vi "ConfigInstr.vi"(6 "InstrumentName":string, 7 "VisaRessIn":refnum<visa-resource-name>, 8 "error in (no error)":errorcluster caption="entrée d'erreur (pas d'erreur)", 9 "FirstClassInst":bool, 10 "Function":string, 11 "GenData In":refnum<class "Calculations.lvclass"> caption="DNL_LabVIEW Object in") -> (0 "error out":errorcluster caption="sortie d'erreur", 3 "GenData Out":refnum<class "Calculations.lvclass"> caption="DNL_LabVIEW Object out")   [LabVIEW 2019, in "Calculations.lvclass"]
uses:
  Calculations.lvclass
  C:/Programmes Labview/LabScanV1A/DevicesClass/BaseDevice/BaseDevice.lvclass
  DefaultDev_Func.ctl
  Calculations.lvclass/Calculations.ctl
  DevicesClass/BaseDevice/BaseDevice.lvclass/BaseDevice.ctl
  DevicesClass/BaseDevice/Accessor/SetShowInstrNm.vi
panel:
  in  "Class_Func":T1
  out "VisaRessOut":refnum<visa-resource-name>
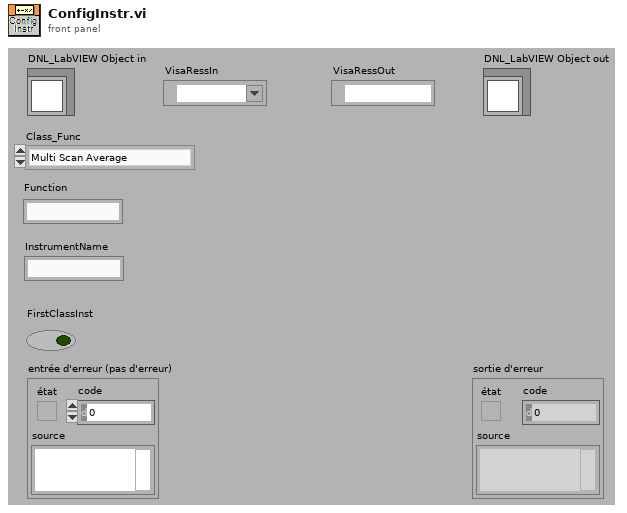
[diagram p1: front panel]
types:
  T1 = typedef "Calculations.lvclass/DefaultDev_Func.ctl" = enum16{"Multi Scan Average", "Running Average", "Summ"}
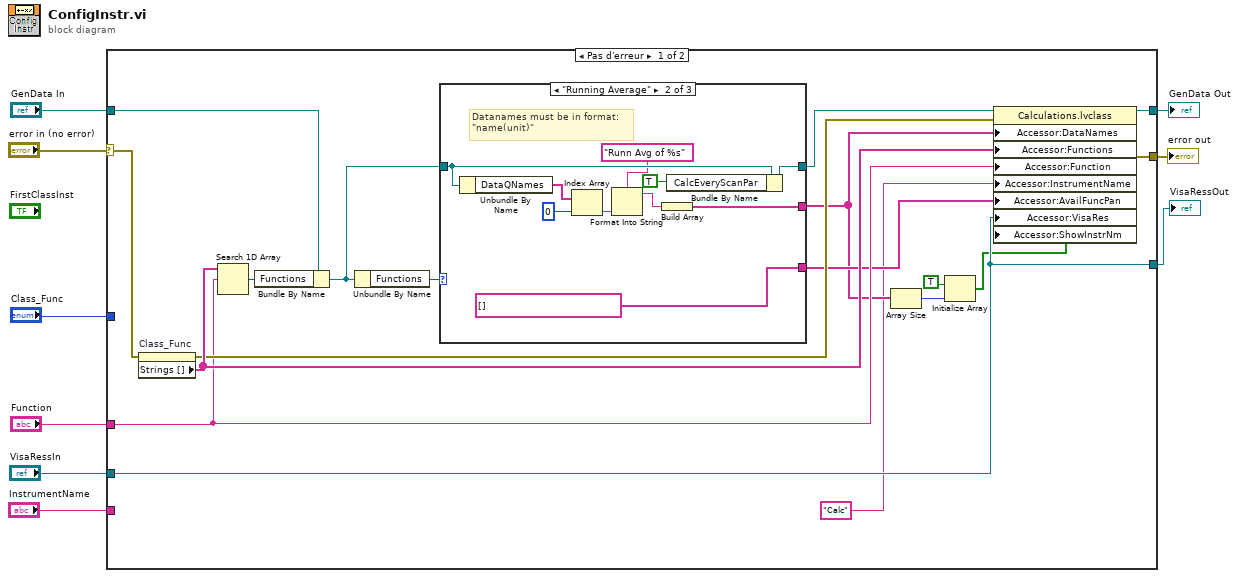
[diagram p0: block diagram]
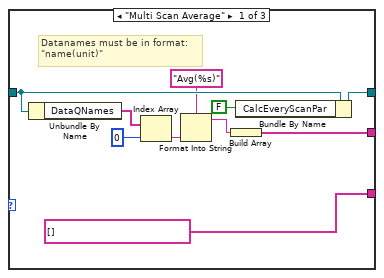
[diagram p2: hidden frame]
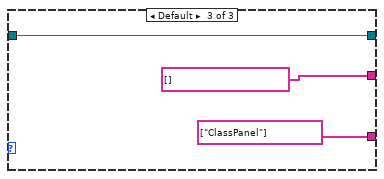
[diagram p3: hidden frame]
diagram:
  n1 = case shown="Pas d'erreur" "error in (no error)" {
    selector: "error in (no error)" -> [w21 w52]
    tunnel: [w27 w52] -> w8
    tunnel: "GenData In" -> [w22 w51]
    tunnel: [w26 w51] -> w6
    tunnel: "Class_Func" -> [_ _]
    tunnel: "Function" -> [w17 _]
    tunnel: "InstrumentName" -> [_ _]
    tunnel: "VisaRessIn" -> [w15 _]
    tunnel: [w15 _] -> w1
    frame No Error {
      n2 = property on="Class_Func" class="Énum (strict)"(error in=w21) -> (error out=w20:errorcluster, "Strings []"=w24:string[])  [unwired: 1 in, 1 out]
      n3 = Search 1D Array(1D array=w24, element=w17) -> (index of element=w23:i32)  [unwired: 1 in]
      n4 = Bundle By Name(cluster=w22, "Functions"=w23) -> (w19:refnum<class "Calculations.lvclass">)
      n5 = Unbundle By Name(w19) -> ("Functions"=w25:T1)
      n6 = case shown="\"Running Average\"" w25 {
        tunnel: [w30 w40 string[] []] -> w12
        tunnel: w19 -> [w36 w46 w49]
        tunnel: [w29 w39 w49] -> w18
        tunnel: [string[] [] string[] [] string[] ["ClassPanel"]] -> w16
        frame "Multi Scan Average" {
          # "Datanames must be in format:\n\"name(unit)\""
          n7 = Unbundle By Name(w36) -> ("DataQNames"=w34:string[])
          n8 = Index Array(array=w34, index=0) -> (element=w33:string)
          n9 = Format Into String(format string="Avg(%s)", w33) -> (resulting string=w31:string)  [unwired: 2 in, 1 out]
          n10 = Build Array(w31) -> (w30:string[])
          n11 = Bundle By Name(cluster=w36, "CalcEveryScanPar"=FALSE) -> (w29:refnum<class "Calculations.lvclass">)
        }
        frame "Running Average" {
          # "Datanames must be in format:\n\"name(unit)\""
          n12 = Unbundle By Name(w46) -> ("DataQNames"=w44:string[])
          n13 = Index Array(array=w44, index=0) -> (element=w43:string)
          n14 = Format Into String(format string="Runn Avg of %s", w43) -> (resulting string=w41:string)  [unwired: 2 in, 1 out]
          n15 = Build Array(w41) -> (w40:string[])
          n16 = Bundle By Name(cluster=w46, "CalcEveryScanPar"=TRUE) -> (w39:refnum<class "Calculations.lvclass">)
        }
        frame Default {
        }
      }
      n17 = Array Size(array=w12) -> (size(s)=w14:i32)
      n18 = Initialize Array(TRUE, w14) -> (w11:bool[])
      n19 = property class="Calculations.lvclass"(reference=w18, error in=w20, "Accessor:DataNames"=w12, "Accessor:Functions"=w24, "Accessor:Function"=w17, "Accessor:InstrumentName"="Calc" ("InstrumentName"), "Accessor:AvailFuncPan"=w16, "Accessor:VisaRes"=w15, "Accessor:ShowInstrNm"=w11) -> (reference out=w26:refnum<class "Calculations.lvclass">, error out=w27:errorcluster)
    }
    frame Error {
    }
  }
  "error out" <- w8
  "GenData Out" <- w6
  "VisaRessOut" <- w1
